vi "Parse DI Cmd.vi"(10 "FIFO Indexes":T6={"Mode"=0, "Digital Input"=0, "Default Profile Index"=0, "Cal Freq [Hz]"=0, "Cal Duration [s]"=0, "Cal Increment [s]"=0, "Cal Pulses"=-1, "TMP Command Sequence"=[], "EPT TDC Offset [CAD]"=0, "EPT Window Start [DBTDC]"=0, "EPT Window End [DBTDC]"=0, "EPT Angles"=[], "EPT Skip Fire"=0, "EPT Skip Index"=0, "EPT Precharge Duration [s]"=-1, "EPT Precharge Profile Index"=-1}, 11 "Device Inputs":dbl[](array[numeric])) -> (3 "Injection Setup out":T1 {"EPT Precharge Profile Index" max=15; "EPT Precharge Duration [s]" min=0 format="%#_4p"; "Default Profile Index" max=15; "Cal Increment [s]" format="%#_3p"; "TMP Command Sequence"."Profile Index" max=7; "TMP Command Sequence"."Duration [s]" min=0 max=100 format="%#_3p"; "Cal Pulses" max=511; "EPT Skip Index" max=7; "EPT Angles"."Profile Index" max=7; "EPT Angles"."Duration [s]" min=0 max=100 format="%#_3p"; "Cal Duration [s]" format="%#_3p"; "Cal Freq [Hz]" format="%#_3p"})   [LabVIEW 2016, in "DCM Engine.lvlib"]
uses:
  DCM Engine.lvlib
  Shared/Types/DI Command Indexes.ctl
  Built/DCM Classes Packed/Pharlap/C/DCM-Classes.lvlibp/DCM/DI/RT/Command.ctl
  Built/DCM Classes Packed/Pharlap/C/DCM-Classes.lvlibp/1abvi3w/vi.lib/Powertrain Controls/Device Drivers/DCM/DI/FPGA/Mode.ctl
  Built/DCM Classes Packed/Pharlap/C/DCM-Classes.lvlibp/1abvi3w/vi.lib/Powertrain Controls/Device Drivers/DCM/Rev0/FPGA/Digital Channel.ctl
  Built/DCM Classes Packed/Pharlap/C/DCM-Classes.lvlibp/DCM/DI/RT/Command Sequence.ctl
  Built/DCM Classes Packed/Pharlap/C/DCM-Classes.lvlibp/DCM/DI/RT/Angle Control.ctl
  Built/DCM Classes Packed/Pharlap/C/DCM-Classes.lvlibp/1abvi3w/vi.lib/Powertrain Controls/Device Drivers/DCM/DI/FPGA/DCM - FPGA - DI.lvlib
  Built/DCM Classes Packed/Pharlap/C/DCM-Classes.lvlibp/1abvi3w/vi.lib/Powertrain Controls/Device Drivers/DCM/Rev0/FPGA/DCM - FPGA.lvlib
  Built/DCM Classes Packed/Pharlap/C/DCM-Classes.lvlibp/DCM/DI/RT/DCM - RT - DI.lvlib
  DCM Shared.lvlib
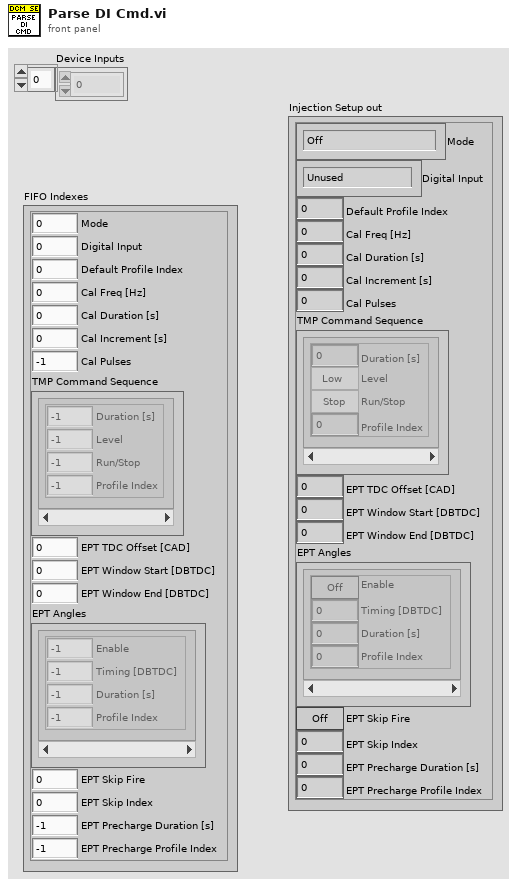
[diagram p1: front panel]
types:
  T1 = typedef "DCM-Classes.lvlibp/DCM - RT - DI.lvlib/Command.ctl" = cluster{"Mode":T2, "Digital Input":T3, "Default Profile Index":u8, "Cal Freq [Hz]":sgl, "Cal Duration [s]":sgl, "Cal Increment [s]":sgl, "Cal Pulses":u16, "TMP Command Sequence":T4[], "EPT TDC Offset [CAD]":sgl, "EPT Window Start [DBTDC]":sgl, "EPT Window End [DBTDC]":sgl, "EPT Angles":T5[], "EPT Skip Fire":bool, "EPT Skip Index":u8, "EPT Precharge Duration [s]":sgl, "EPT Precharge Profile Index":u8}
  T2 = typedef "DCM-Classes.lvlibp/DCM - FPGA - DI.lvlib/Mode.ctl" = enum8{"Off", "Direct", "Calibration", "Triggered Multi-Pulse", "Engine Position Tracking"}
  T3 = typedef "DCM-Classes.lvlibp/DCM - FPGA.lvlib/Digital Channel.ctl" = enum8{"Unused", "User OS", "Diff IO 1", "Diff IO 2", "Diff IO 3", "Diff IO 4", "Diff IO 5", "Diff IO 6", "Diff IO 7", "Diff IO 8", "Aux 1", "Aux 2", "Aux 3", "Aux 4", "Aux 5", "Aux 6", "Aux 7", "Aux 8", "Aux 9", "Aux 10", "Aux 11", "Aux 12", "Aux 13", "Aux 14", "Aux 15", "Aux 16"}
  T4 = typedef "DCM-Classes.lvlibp/DCM - RT - DI.lvlib/Command Sequence.ctl" = cluster{"Duration [s]":sgl, "Level":bool, "Run/Stop":bool, "Profile Index":u8}
  T5 = typedef "DCM-Classes.lvlibp/DCM - RT - DI.lvlib/Angle Control.ctl" = cluster{"Enable":bool, "Timing [DBTDC]":sgl, "Duration [s]":sgl, "Profile Index":u8}
  T6 = typedef "DCM Shared.lvlib/DI Command Indexes.ctl" = cluster{"Mode":i32, "Digital Input":i32, "Default Profile Index":i32, "Cal Freq [Hz]":i32, "Cal Duration [s]":i32, "Cal Increment [s]":i32, "Cal Pulses":i32, "TMP Command Sequence":cluster{"Duration [s]":i32, "Level":i32, "Run/Stop":i32, "Profile Index":i32}[], "EPT TDC Offset [CAD]":i32, "EPT Window Start [DBTDC]":i32, "EPT Window End [DBTDC]":i32, "EPT Angles":cluster{"Enable":i32, "Timing [DBTDC]":i32, "Duration [s]":i32, "Profile Index":i32}[], "EPT Skip Fire":i32, "EPT Skip Index":i32, "EPT Precharge Duration [s]":i32, "EPT Precharge Profile Index":i32}
  T7 = cluster{"Duration [s]":i32, "Level":i32, "Run/Stop":i32, "Profile Index":i32}[]
  T8 = cluster{"Enable":i32, "Timing [DBTDC]":i32, "Duration [s]":i32, "Profile Index":i32}[]
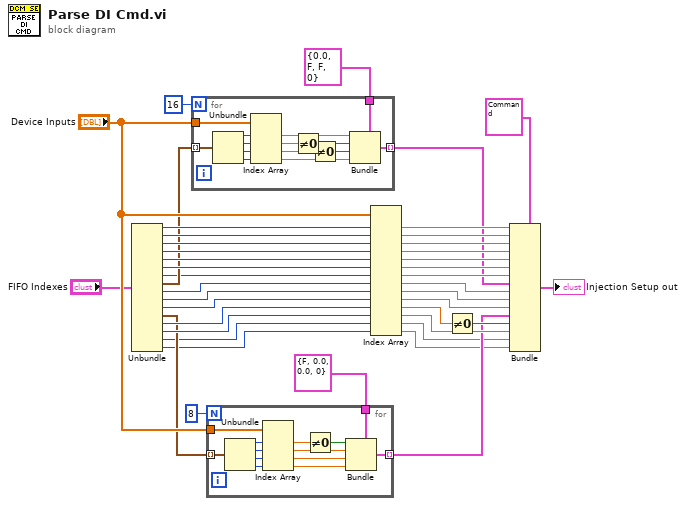
[diagram p0: block diagram]
diagram:
  n1 = Unbundle("FIFO Indexes") -> ("Mode"=w26:i32, "Digital Input"=w27:i32, "Default Profile Index"=w28:i32, "Cal Freq [Hz]"=w29:i32, "Cal Duration [s]"=w30:i32, "Cal Increment [s]"=w18:i32, "Cal Pulses"=w13:i32, "TMP Command Sequence"=w14:T7, "EPT TDC Offset [CAD]"=w31:i32, "EPT Window Start [DBTDC]"=w17:i32, "EPT Window End [DBTDC]"=w15:i32, "EPT Angles"=w16:T8, "EPT Skip Fire"=w32:i32, "EPT Skip Index"=w23:i32, "EPT Precharge Duration [s]"=w4:i32, "EPT Precharge Profile Index"=w3:i32)
  n2 = for {
    N: 16 -> [_]
    tunnel: w14 -> [w53] mode=indexing
    tunnel: T4 {"Duration [s]"=0.0, "Level"=FALSE, "Run/Stop"=FALSE, "Profile Index"=0} ("Command") -> [w55]
    tunnel: [w54] -> w11 mode=indexing
    tunnel: "Device Inputs" -> [w48]
    n3 = Unbundle(w53) -> ("Duration [s]"=w52:i32, "Level"=w51:i32, "Run/Stop"=w50:i32, "Profile Index"=w49:i32)
    n4 = Index Array(array=w48, index #1=w52, index #2=w51, index #3=w50, index #4=w49) -> (element #1=w47:dbl, element #2=w46:dbl, element #3=w44:dbl, element #4=w42:dbl)
    n5 = Not Equal To 0?(x=w46) -> (x != 0?=w45:bool)
    n6 = Not Equal To 0?(x=w44) -> (x != 0?=w43:bool)
    n7 = Bundle(cluster=w55, "Duration [s]"=w47, "Level"=w45, "Run/Stop"=w43, "Profile Index"=w42) -> (w54:T4)
  }
  n8 = for {
    N: 8 -> [_]
    tunnel: w16 -> [w67] mode=indexing
    tunnel: [w68] -> w8 mode=indexing
    tunnel: "Device Inputs" -> [w62]
    tunnel: T5 {"Enable"=FALSE, "Timing [DBTDC]"=0.0, "Duration [s]"=0.0, "Profile Index"=0} ("Injection Control") -> [w56]
    n9 = Unbundle(w67) -> ("Enable"=w66:i32, "Timing [DBTDC]"=w65:i32, "Duration [s]"=w64:i32, "Profile Index"=w63:i32)
    n10 = Index Array(array=w62, index #1=w66, index #2=w65, index #3=w64, index #4=w63) -> (element #1=w61:dbl, element #2=w58:dbl, element #3=w59:dbl, element #4=w57:dbl)
    n11 = Not Equal To 0?(x=w61) -> (x != 0?=w60:bool)
    n12 = Bundle(cluster=w56, "Enable"=w60, "Timing [DBTDC]"=w58, "Duration [s]"=w59, "Profile Index"=w57) -> (w68:T5)
  }
  n13 = Index Array(array="Device Inputs", index #1=w26, index #2=w27, index #3=w28, index #4=w29, index #5=w30, index #6=w18, index #7=w13, index #8=w31, index #9=w17, index #10=w15, index #11=w32, index #12=w23, index #13=w4, index #14=w3) -> (element #1=w33:dbl, element #2=w34:dbl, element #3=w35:dbl, element #4=w36:dbl, element #5=w37:dbl, element #6=w19:dbl, element #7=w12:dbl, element #8=w20:dbl, element #9=w21:dbl, element #10=w7:dbl, element #11=w9:dbl, element #12=w22:dbl, element #13=w6:dbl, element #14=w5:dbl)
  n14 = Not Equal To 0?(x=w9) -> (x != 0?=w10:bool)
  n15 = Bundle(cluster=T1 {"Mode"=enum."Off", "Digital Input"=enum."Unused", "Default Profile Index"=0, "Cal Freq [Hz]"=0.0, "Cal Duration [s]"=0.0, "Cal Increment [s]"=0.0, "Cal Pulses"=0, "TMP Command Sequence"=[{"Duration [s]"=0.0, "Level"=FALSE, "Run/Stop"=FALSE, "Profile Index"=0}, {"Duration [s]"=0.0, "Level"=FALSE, "Run/Stop"=FALSE, "Profile Index"=0}, {"Duration [s]"=0.0, "Level"=FALSE, "Run/Stop"=FALSE, "Profile Index"=0}, {"Duration [s]"=0.0, "Level"=FALSE, "Run/Stop"=FALSE, "Profile Index"=0}, {"Duration [s]"=0.0, "Level"=FALSE, "Run/Stop"=FALSE, "Profile Index"=0}, {"Duration [s]"=0.0, "Level"=FALSE, "Run/Stop"=FALSE, "Profile Index"=0}, {"Duration [s]"=0.0, "Level"=FALSE, "Run/Stop"=FALSE, "Profile Index"=0}, {"Duration [s]"=0.0, "Level"=FALSE, "Run/Stop"=FALSE, "Profile Index"=0}], "EPT TDC Offset [CAD]"=0.0, "EPT Window Start [DBTDC]"=0.0, "EPT Window End [DBTDC]"=0.0, "EPT Angles"=[{"Enable"=FALSE, "Timing [DBTDC]"=0.0, "Duration [s]"=0.0, "Profile Index"=0}, {"Enable"=FALSE, "Timing [DBTDC]"=0.0, "Duration [s]"=0.0, "Profile Index"=0}, {"Enable"=FALSE, "Timing [DBTDC]"=0.0, "Duration [s]"=0.0, "Profile Index"=0}, {"Enable"=FALSE, "Timing [DBTDC]"=0.0, "Duration [s]"=0.0, "Profile Index"=0}], "EPT Skip Fire"=FALSE, "EPT Skip Index"=0, "EPT Precharge Duration [s]"=0.0, "EPT Precharge Profile Index"=0}, "Mode"=w33, "Digital Input"=w34, "Default Profile Index"=w35, "Cal Freq [Hz]"=w36, "Cal Duration [s]"=w37, "Cal Increment [s]"=w19, "Cal Pulses"=w12, "TMP Command Sequence"=w11, "EPT TDC Offset [CAD]"=w20, "EPT Window Start [DBTDC]"=w21, "EPT Window End [DBTDC]"=w7, "EPT Angles"=w8, "EPT Skip Fire"=w10, "EPT Skip Index"=w22, "EPT Precharge Duration [s]"=w6, "EPT Precharge Profile Index"=w5) -> (→"Injection Setup out":T1)
